vi "Send Software Trigger.vi"(8 "error in (no error)":errorcluster {"code" format="%.0x"}, 11 "VISA resource name":refnum<visa-resource-name>) -> (0 "error out":errorcluster {"code" format="%.0x"}, 3 "VISA resource name out":refnum<visa-resource-name>)   [LabVIEW 2014, in "Agilent N6700 Series.lvlib"]
doc: "Sends trigger signal to trigger the power supply. Call this VI if you configure the power supply to respond to software triggers. To use this VI please configure trigger source to Software in <B>Configure Trigger Source.vi</B>"
uses:
  Agilent N6700 Series.lvlib
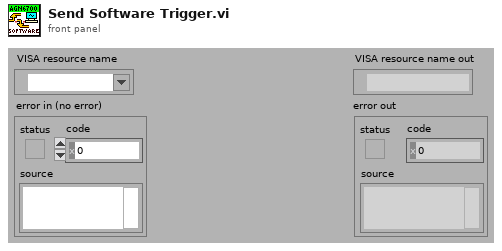
[diagram p1: front panel]
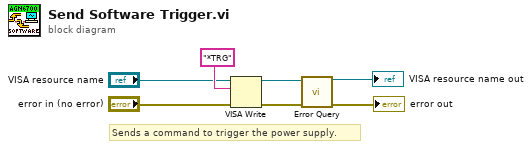
[diagram p0: block diagram]
diagram:
  # "Sends a command to trigger the power supply."
  n1 = VISA Write(VISA resource name="VISA resource name", write buffer="*TRG", error in (no error)="error in (no error)") -> (VISA resource name out=w2:refnum<visa-resource-name>, error out=w1:errorcluster)  [unwired: 1 out]
  n2 = call "Error Query.vi"("VISA resource name"=w2, "error in (no error)"=w1) -> ("VISA resource name out"=→"VISA resource name out":refnum<visa-resource-name>, "error out"=→"error out":errorcluster)  [unwired: 10 in, 2 out]
